vi "GlobalPosYbyTime.vi"() -> ()   [LabVIEW 2022 SP3]
panel:
  out "Array":dbl[](array[numeric])
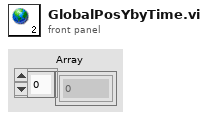
[diagram p1: front panel]
diagram:
